vi "Day 12 Task 2 no recurse.vi"() -> ()   [LabVIEW 2018]
uses:
  Cave Info1.ctl
  <userlib>/_OpenG.lib/array/array.llb/Search 1D Array (String)__ogtk.vi
  <userlib>/_OpenG.lib/array/array.llb/Remove Duplicates from 1D Array (String)__ogtk.vi
panel:
  out "size(s)":i32
  out "Valid paths found":cluster{"Path":string[]}[](array[cluster])
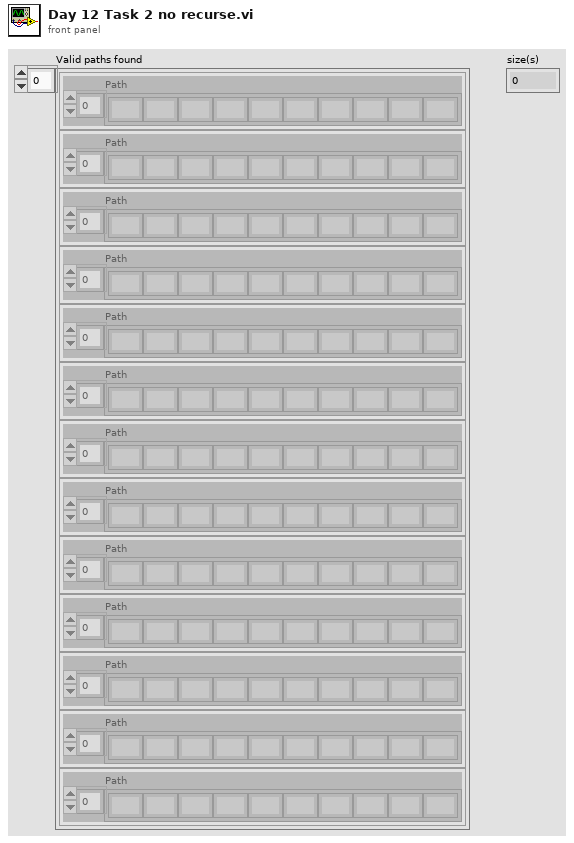
[diagram p1: front panel]
types:
  T1 = typedef "Cave Info1.ctl" = cluster{"Cave":string, "Is small?":bool, "Connections":string[]}
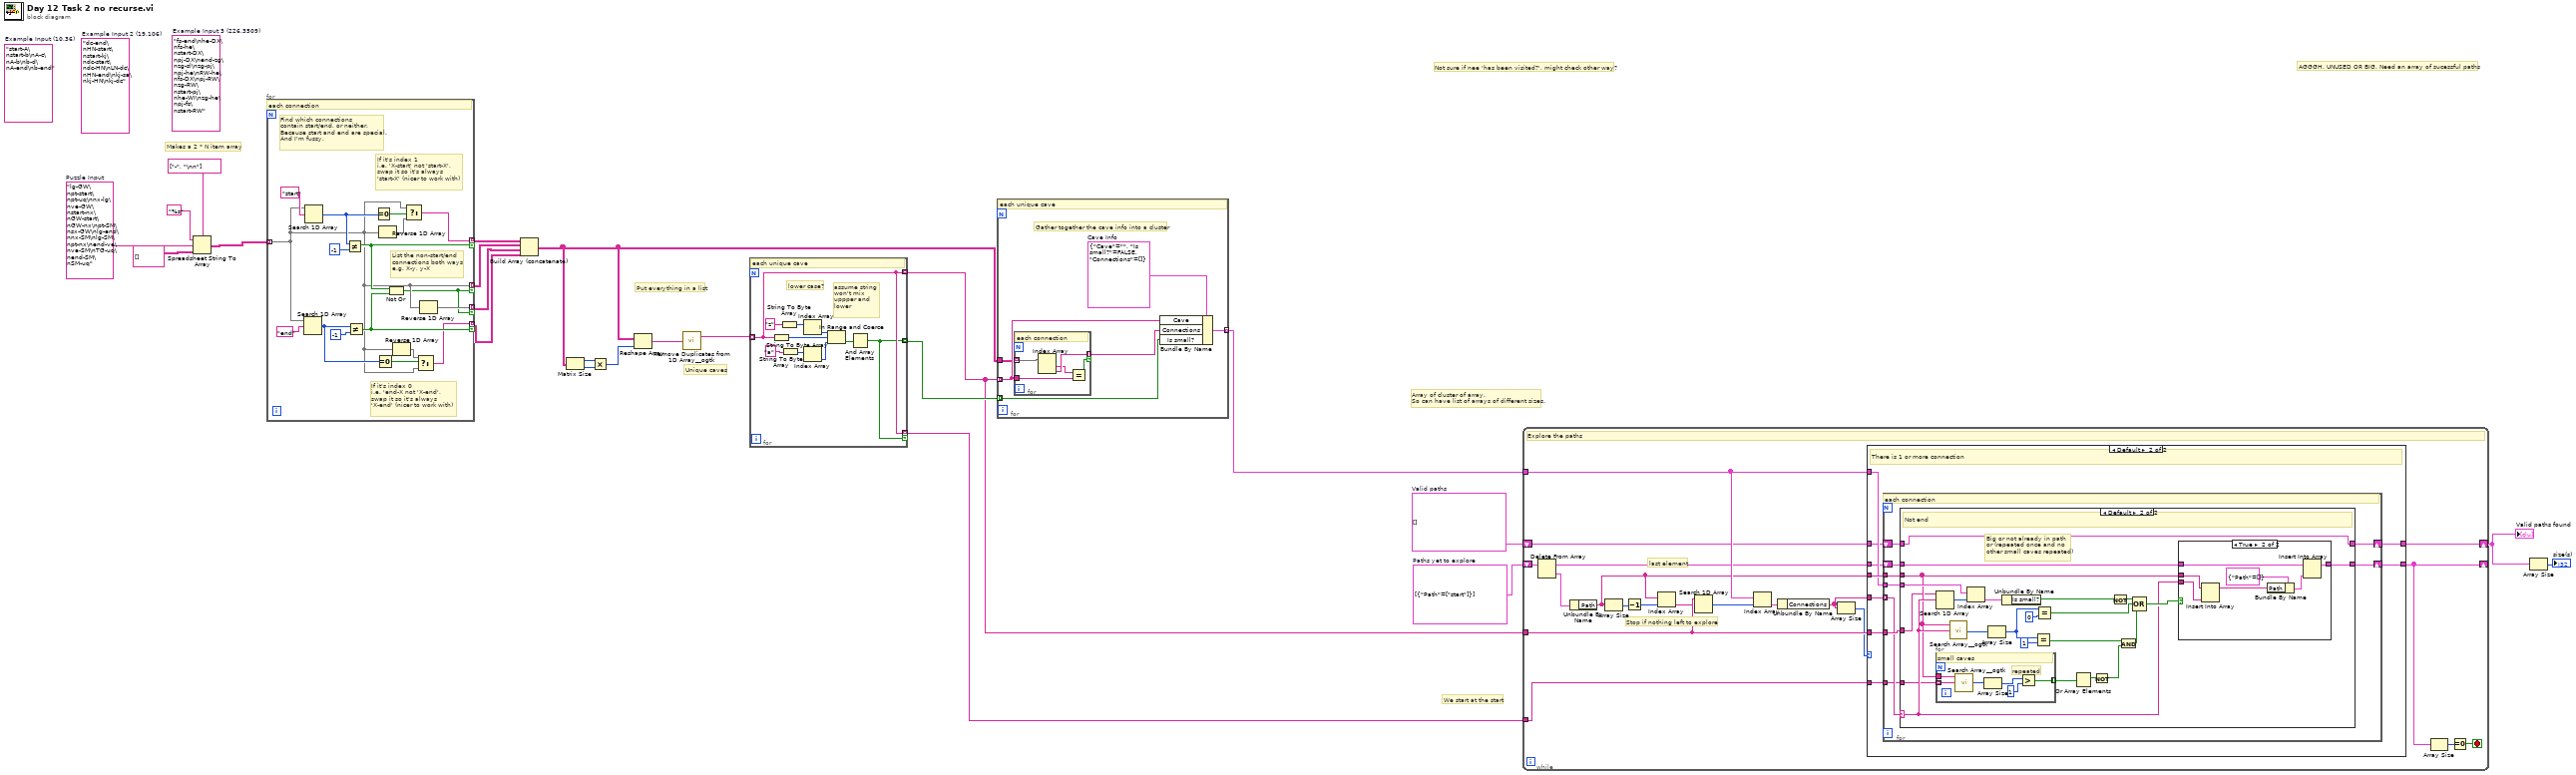
[diagram p0: block diagram]
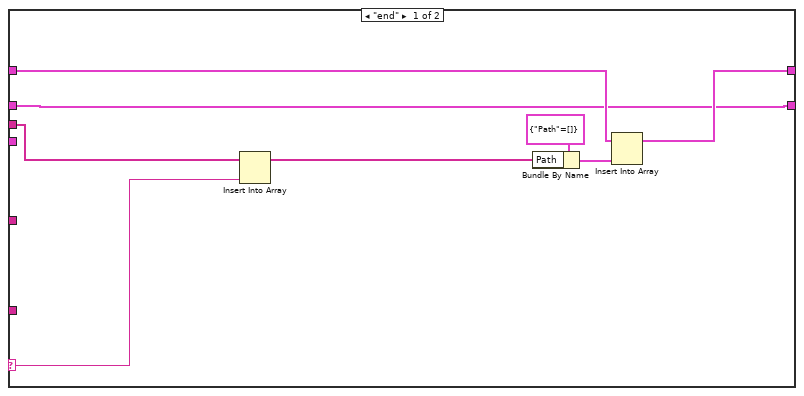
[diagram p3: hidden frame]
diagram:
  w8 = cluster{"Path":string[]}[] []  # Valid paths
  w10 = cluster{"Path":string[]}[] [{"Path"=["start"]}]  # Paths yet to explore
  (unwired) "fs-end\nhe-DX\nfs-he\nstart-DX\npj-DX\nend-zg\nzg-sl\nzg-pj\npj-he\nRW-he\nfs-DX\npj-RW\nzg-RW\nstart-pj\nhe-WI\nzg-he\npj-fs\nstart-RW"  # Example Input 3 (226,3509)
  (unwired) "dc-end\nHN-start\nstart-kj\ndc-start\ndc-HN\nLN-dc\nHN-end\nkj-sa\nkj-HN\nkj-dc"  # Example Input 2 (19,106)
  w1 = "lg-GW\npt-start\npt-uq\nnx-lg\nve-GW\nstart-nx\nGW-start\nGW-nx\npt-SM\nsx-GW\nlg-end\nnx-SM\nlg-SM\npt-nx\nend-ve\nve-SM\nTG-uq\nend-SM\nSM-uq"  # Puzzle Input
  (unwired) "start-A\nstart-b\nA-c\nA-b\nb-d\nA-end\nb-end"  # Example Input (10,36)
  # "We start at the start"
  # "Put everything in a list"
  # "Array of cluster of array.\nSo can have list of arrays of different sizes."
  # "AGGGH. UNUSED OR BIG. Need an array of sucessful paths"
  # "Not sure if nee 'has been visited?', might check other way?"
  # "Unique caves"
  # "Makes a 2 * N item array"
  n1 = Spreadsheet String To Array(delimiter (Tab)=string[] ["-", "\nn"], format string="%s", spreadsheet string=w1, array type (2D Dbl)=string[][] []) -> (array=w16:string[][])
  n2 = for {
    tunnel: w16 -> [w26] mode=indexing
    tunnel: [w31] -> w15 mode=indexing if=w36
    tunnel: [w28] -> w12 mode=indexing if=w35
    tunnel: [w26] -> w14 mode=indexing if=w24
    tunnel: [w25] -> w13 mode=indexing if=w24
    # "List the non-start/end\nconnections both ways\ne.g. X-y, y-X"
    # "If it's index 0\ni.e. 'end-X not 'X-end',\nswap it so it's always \n'X-end' (nicer to work with)"
    # "Find which connections\ncontain start/end, or neither.\nBecause start and end are special.\nAnd I'm fussy."
    # "If it's index 1\ni.e. 'X-start' not 'start-X',\nswap it so it's always \n'start-X' (nicer to work with)"
    # "each connection"
    n3 = Search 1D Array(1D array=w26, element="end") -> (index of element=w27:i32)  [unwired: 1 in]
    n4 = Search 1D Array(1D array=w26, element="start") -> (index of element=w34:i32)  [unwired: 1 in]
    n5 = Not Equal?(x=w34, y=-1) -> (x != y?=w36:bool)
    n6 = Not Equal?(x=w27, y=-1) -> (x != y?=w35:bool)
    n7 = Equal To 0?(x=w34) -> (x = 0?=w33:bool)
    n8 = Equal To 0?(x=w27) -> (x = 0?=w30:bool)
    n9 = Reverse 1D Array(array=w26) -> (reversed array=w32:string[])
    n10 = Not Or(1:w35, 2:w36) -> (0:w24:bool)
    n11 = Reverse 1D Array(array=w26) -> (reversed array=w29:string[])
    n12 = Select(t=w26, s=w33, f=w32) -> (s? t:f=w31:string[])
    n13 = Select(t=w29, s=w30, f=w26) -> (s? t:f=w28:string[])
    n14 = Reverse 1D Array(array=w26) -> (reversed array=w25:string[])
  }
  n15 = Build Array (concatenate)(w15, w14, w13, w12) -> (w5:string[][])
  n16 = Matrix Size(0:w5) -> (1:w19:i32, 2:w20:i32)
  n17 = Multiply(x=w19, y=w20) -> (x*y=w18:i32)
  n18 = Reshape Array(w5, w18) -> (w17:string[])
  n19 = call-poly <userlib>:"Remove Duplicates from 1D Array__ogtk.vi"("Input Array"=w17) -> ("Output Array"=w4:string[])  [unwired: 1 out]
  n20 = for {
    tunnel: w4 -> [w42] mode=indexing
    tunnel: [w42] -> w3 mode=indexing
    tunnel: [w41] -> w11 mode=indexing
    tunnel: [w42] -> w2 mode=indexing if=w41
    # "lower case?"
    # "assume string \nwon't mix\nuppper and\nlower"
    # "each unique cave"
    n21 = String To Byte Array(string=w42) -> (unsigned byte array=w50:u8[])
    n22 = String To Byte Array(string="z" ("format string")) -> (unsigned byte array=w48:u8[])
    n23 = String To Byte Array(string="a" ("format string")) -> (unsigned byte array=w46:u8[])
    n24 = Index Array(array=w48) -> (element=w47:u8)  [unwired: 1 in]
    n25 = Index Array(array=w46) -> (element=w44:u8)  [unwired: 1 in]
    n26 = In Range and Coerce(upper limit=w47, x=w50, lower limit=w44) -> (In Range?=w43:bool[])  [unwired: 1 out]
    n27 = And Array Elements(Boolean array=w43) -> (logical AND=w41:bool)
  }
  n28 = for {
    tunnel: w3 -> [w55] mode=indexing
    tunnel: w5 -> [w52]
    tunnel: [w53] -> w9 mode=indexing
    tunnel: w11 -> [w51] mode=indexing
    w56 = T1 {"Cave"="", "Is small?"=FALSE, "Connections"=[]}  # Cave Info
    # "Gather together the cave info into a cluster"
    # "each unique cave"
    n29 = for {
      tunnel: w55 -> [w61]
      tunnel: [w59] -> w54 mode=indexing if=w60
      tunnel: w52 -> [w57] mode=indexing
      # "each connection"
      n30 = Index Array(array=w57) -> (element #1=w58:string, element #2=w59:string)  [unwired: 2 in]
      n31 = Equal?(x=w58, y=w61) -> (x = y?=w60:bool)
    }
    n32 = Bundle By Name(cluster=w56, "Cave"=w55, "Connections"=w54, "Is small?"=w51) -> (w53:T1)
  }
  n33 = while {
    tunnel: w3 -> [w78]
    tunnel: w9 -> [w77]
    shift-right: [w64] -> _
    shift-left: w10 -> [w67]
    shift-right: [w63] -> w7
    shift-left: w8 -> [w76]
    tunnel: w2 -> [w62]
    stop <- w80 stop-if-true
    # "last element"
    # "Stop if nothing left to explore"
    # "Explore the paths"
    n34 = Delete From Array(array=w67) -> (deleted portion=w66:cluster{"Path":string[]}, array with subset deleted=w65:cluster{"Path":string[]}[])  [unwired: 2 in]
    n35 = Unbundle By Name(w66) -> ("Path"=w70:string[])
    n36 = Array Size(array=w70) -> (size(s)=w75:i32)
    n37 = Decrement(x=w75) -> (x-1=w74:i32)
    n38 = Index Array(array=w70, index=w74) -> (element=w73:string)
    n39 = Search 1D Array(1D array=w78, element=w73) -> (index of element=w72:i32)  [unwired: 1 in]
    n40 = Index Array(array=w77, index=w72) -> (element=w71:T1)
    n41 = Unbundle By Name(w71) -> ("Connections"=w69:string[])
    n42 = Array Size(array=w69) -> (size(s)=w68:i32)
    n43 = case shown="Default" w68 {
      tunnel: w70 -> [_ w91]
      tunnel: w78 -> [_ w90]
      tunnel: w77 -> [_ w89]
      tunnel: w76 -> [w82 w88]
      tunnel: [w82 w87] -> w63
      tunnel: w69 -> [_ w86]
      tunnel: w65 -> [w81 w85]
      tunnel: [w81 w84] -> w64
      tunnel: w62 -> [_ w83]
      frame 0 {
        # "No more connections,\nlet it unqueue the next thing"
      }
      frame Default {
        # "There is 1 or more connection"
        n44 = for {
          tunnel: w86 -> [w97] mode=indexing
          tunnel: w91 -> [w100]
          tunnel: w90 -> [w99]
          tunnel: w89 -> [w98]
          shift-right: [w95] -> w87
          shift-left: w88 -> [w96]
          shift-right: [w93] -> w84
          shift-left: w85 -> [w94]
          tunnel: w83 -> [w92]
          # "each connection"
          n45 = case shown="Default" w97 {
            selector: w97 -> [w108 w119]
            tunnel: w100 -> [w102 w118]
            tunnel: w99 -> [_ w117]
            tunnel: w98 -> [_ w130]
            tunnel: w96 -> [w107 w128]
            tunnel: [w103 w128] -> w95
            tunnel: w94 -> [w101 w124]
            tunnel: [w101 w123] -> w93
            tunnel: w92 -> [_ w112]
            frame "end" {
              n46 = Insert Into Array(array=w102, new element=w108) -> (w105:string[])  [unwired: 1 in]
              n47 = Bundle By Name(cluster=cluster{"Path":string[]} {"Path"=[]} ("new element/subarray"), "Path"=w105) -> (w104:cluster{"Path":string[]})
              n48 = Insert Into Array(array=w107, new element=w104) -> (w103:cluster{"Path":string[]}[])  [unwired: 1 in]
            }
            frame Default {
              # "Big or not already in path\nor (repeated once and no\nother small caves repeated)"
              # "Not end"
              n49 = Search 1D Array(1D array=w117, element=w119) -> (index of element=w131:i32)  [unwired: 1 in]
              n50 = for {
                tunnel: w118 -> [w137]
                tunnel: w112 -> [w134] mode=indexing
                tunnel: [w132] -> w109 mode=indexing
                # "repeated"
                # "small caves"
                n51 = call-poly <userlib>:"Search Array__ogtk.vi"("Array"=w137, "Element Data"=w134) -> ("Indices of Elements"=w136:i32[])  [unwired: 7 in]
                n52 = Array Size(array=w136) -> (size(s)=w135:i32)
                n53 = Greater?(x=w135, y=1 ("x")) -> (0:w132:bool)
              }
              n54 = call-poly <userlib>:"Search Array__ogtk.vi"("Array"=w118, "Element Data"=w119) -> ("Indices of Elements"=w120:i32[])  [unwired: 7 in]
              n55 = Index Array(array=w130, index=w131) -> (element=w129:T1)
              n56 = Array Size(array=w120) -> (size(s)=w116:i32)
              n57 = Unbundle By Name(w129) -> ("Is small?"=w127:bool)
              n58 = Equal?(x=w116, y=1) -> (x = y?=w114:bool)
              n59 = Equal?(x=w116, y=0) -> (x = y?=w125:bool)
              n60 = Or Array Elements(Boolean array=w109) -> (logical OR=w110:bool)
              n61 = Not(x=w110) -> (.not. x?=w111:bool)
              n62 = Not(x=w127) -> (.not. x?=w126:bool)
              n63 = And(x=w114, y=w111) -> (x .and. y?=w113:bool)
              n64 = Compound Arithmetic op=OR(w126, w125, w113) -> (w122:bool)
              n65 = case shown="True" w122 {
                tunnel: w118 -> [_ w143]
                tunnel: w119 -> [_ w142]
                tunnel: w124 -> [w138 w141]
                tunnel: [w138 w140] -> w123
                frame False {
                }
                frame True {
                  n66 = Insert Into Array(array=w143, new element=w142) -> (w144:string[])  [unwired: 1 in]
                  n67 = Bundle By Name(cluster=cluster{"Path":string[]} {"Path"=[]} ("new element/subarray"), "Path"=w144) -> (w139:cluster{"Path":string[]})
                  n68 = Insert Into Array(array=w141, new element=w139) -> (w140:cluster{"Path":string[]}[])  [unwired: 1 in]
                }
              }
            }
          }
        }
      }
    }
    n69 = Array Size(array=w64) -> (size(s)=w79:i32)
    n70 = Equal To 0?(x=w79) -> (x = 0?=w80:bool)
  }
  "Valid paths found" <- w7
  n71 = Array Size(array=w7) -> (size(s)=→"size(s)":i32)
